vi "Value Entry_BOOL.vi"(11 "Value In":bool) -> (2 "Apply":bool, 3 "Value Out":bool)   [LabVIEW 2018, in "Tag Watchlist.lvlib"]
doc: "Boolean value pop-up window. Use spacebar to toggle the value."
uses:
  Tag Watchlist.lvlib
panel:
  in  "Cancel":bool
  in  "OK":bool
  in  "New Value":bool
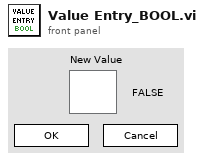
[diagram p1: front panel]
types:
  T1 = typedef "eventvkey.ctl" = enum16{"ASCII", "Enter", "Return", "Shift", "Ctrl", "Alt", "Cmd", "Opt", "Caps", "NumLock", "Clear", "Break", "Up", "Down", "Left", "Right", "Insert", "Delete", "Home", "End", "PageUp", "PageDown", "Escape", "Help", "Pause", "ScrollLock", "F1", "F2", "F3", "F4", "F5", "F6", "F7", "F8", "F9", "F10", "F11", "F12", "F13", "F14", "F15", "F16", "F17", "F18", "F19", "F20", "F21", "F22", "F23", "F24", "Play", "VolumeUp", "VolumeDown", "Mute", "Two Byte Char"}
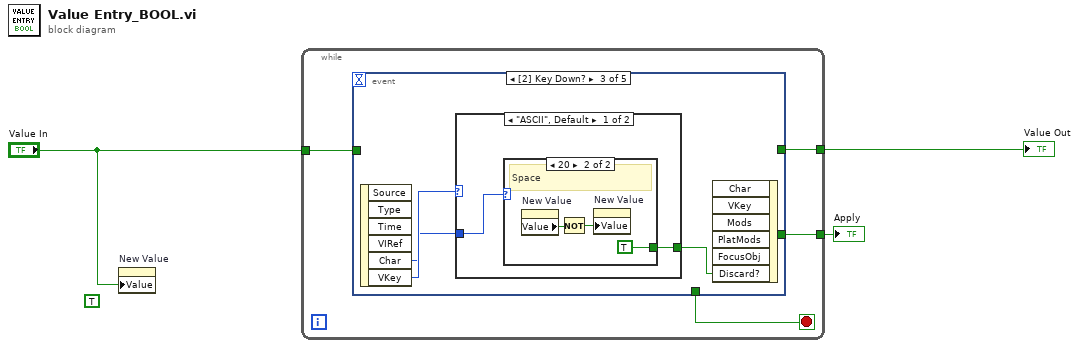
[diagram p0: block diagram]
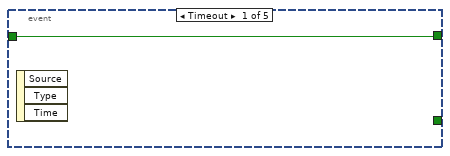
[diagram p2: hidden frame]
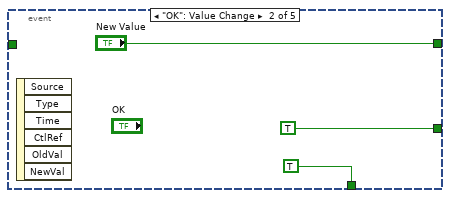
[diagram p3: hidden frame]
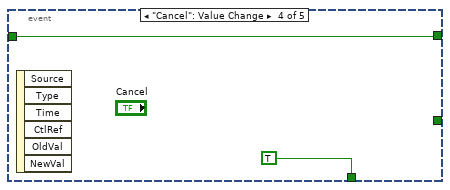
[diagram p6: hidden frame]
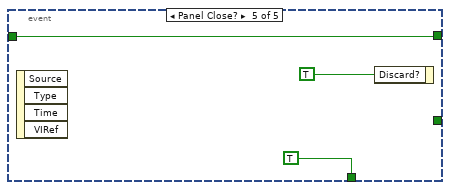
[diagram p7: hidden frame]
diagram:
  (unwired) TRUE ("Key Focus")
  n1 = property on="New Value" class="Bool (strict)"("Value"="Value In") -> ()  [unwired: 2 in, 2 out]
  n2 = while {
    tunnel: "Value In" -> [w7]
    tunnel: [w6] -> w3
    tunnel: [w4] -> w2
    stop <- w5 stop-if-true
    n3 = event shown="[2] Key Down?" {
      selector: _ -> [_ _ _ _ _]
      dyn-events: _ -> [_ _ _ _ _]
      timeout: _ -> [_ _ _ _ _]
      tunnel: w7 -> [w8 _ _ w20 w22]
      tunnel: [w8 "New Value" _ w20 w22] -> w6
      tunnel: [_ TRUE _ TRUE TRUE] -> w5
      tunnel: [_ TRUE _ _ _] -> w4
      event Timeout {
        n4 = event-data() -> ()  [unwired: 1 in, 3 out]
      }
      event "OK": Value Change {
        n5 = event-data() -> ()  [unwired: 1 in, 6 out]
      }
      event Key Down? {
        n6 = event-data() -> ("Char"=w13:i16, "VKey"=w14:T1)  [unwired: 1 in, 4 out]
        n7 = case shown="\"ASCII\", Default" w14 {
          tunnel: w13 -> [w16 _]
          tunnel: [w15 _] -> w12
          frame "ASCII", Default {
            n8 = case shown="20" w16 {
              tunnel: [_ TRUE ("Discard?")] -> w15
              frame 0, Default {
              }
              frame 32 {
                # "Space"
                n9 = property on="New Value" class="Bool (strict)"() -> ("Value"=w19:bool)  [unwired: 2 in, 2 out]
                n10 = Not(x=w19) -> (.not. x?=w18:bool)
                n11 = property on="New Value" class="Bool (strict)"("Value"=w18) -> ()  [unwired: 2 in, 2 out]
              }
            }
          }
          frame "Enter" {
          }
        }
        n12 = event-data("Discard?"=w12) -> ()  [unwired: 6 in, 1 out]
      }
      event "Cancel": Value Change {
        n13 = event-data() -> ()  [unwired: 1 in, 6 out]
      }
      event Panel Close? {
        n14 = event-data() -> ()  [unwired: 1 in, 4 out]
        n15 = event-data("Discard?"=TRUE) -> ()  [unwired: 1 in, 1 out]
      }
    }
  }
  "Value Out" <- w3
  "Apply" <- w2
